vi "JoyCurve.vi"(8 "error in (no error)":errorcluster, 10 "Powers":T2, 11 "Axes":T1) -> (0 "error out":errorcluster, 3 "Axes Out":T1)   [LabVIEW 2014]
doc: "Takes joystick values and raises them to a specified power.\nAllows for fine-tuning of joystick sensitivity.\ni.e. \"screws them around\" -James"
uses:
  JoyCurve Powers.ctl
  JoyCurve Axes.ctl
panel:
  in  "Tab Control":enum32{"Page 1"}(tab)
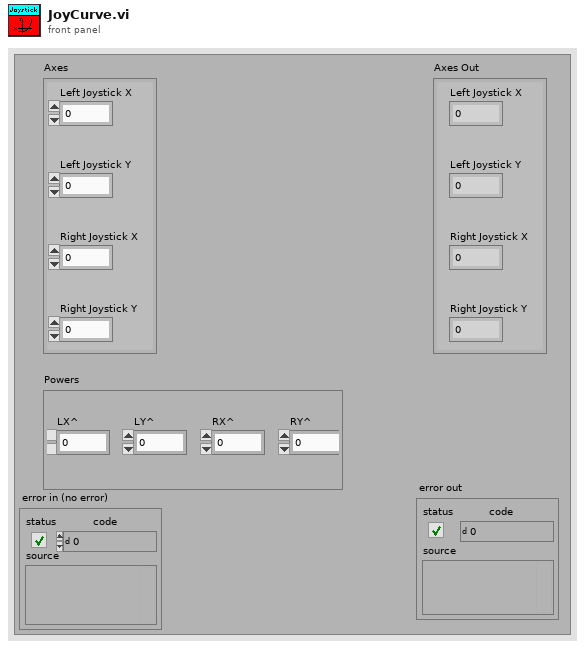
[diagram p1: front panel]
types:
  T1 = typedef "JoyCurve Axes.ctl" = cluster{"Left Joystick X":dbl, "Left Joystick Y":dbl, "Right Joystick X":dbl, "Right Joystick Y":dbl}
  T2 = typedef "JoyCurve Powers.ctl" = cluster{"LX^":dbl, "LY^":dbl, "RX^":dbl, "RY^":dbl}
  T3 = cluster{"[0]":dbl, "[1]":dbl, "[2]":dbl, "[3]":dbl}
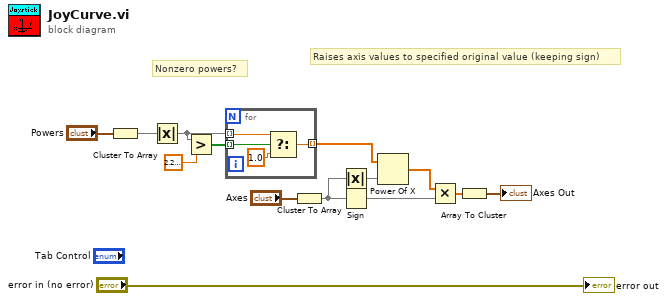
[diagram p0: block diagram]
diagram:
  # "Nonzero powers?"
  # "Raises axis values to specified original value (keeping sign)"
  n1 = Cluster To Array(cluster="Powers") -> (array=w2:dbl[])
  n2 = Absolute Value(x=w2) -> (abs(x)=w1:dbl[])
  n3 = Greater?(x=w1, y=2.220446049250313e-16) -> (0:w4:bool[])
  n4 = for {
    tunnel: w4 -> [w18] mode=indexing
    tunnel: w1 -> [w17] mode=indexing
    tunnel: [w15] -> w3 mode=indexing
    n5 = Select(t=w17, s=w18, f=1.0) -> (s? t:f=w15:dbl)
  }
  n6 = Cluster To Array(cluster="Axes") -> (array=w8:dbl[])
  n7 = Absolute Value(x=w8) -> (abs(x)=w7:dbl[])
  n8 = Sign(1:w8) -> (0:w14:dbl[])
  n9 = Power Of X(1:w7, 2:w3) -> (0:w6:dbl[])
  n10 = Multiply(x=w6, y=w14) -> (x*y=w11:dbl[])
  n11 = Array To Cluster(array=w11) -> (cluster=→"Axes Out":T3)
  "error out" <- "error in (no error)"
